vi "data kontrol.vi"() -> ()   [LabVIEW 2021]
panel:
  out "Array 2":dbl[](array[numeric])
  out "Array":dbl[](array[numeric])
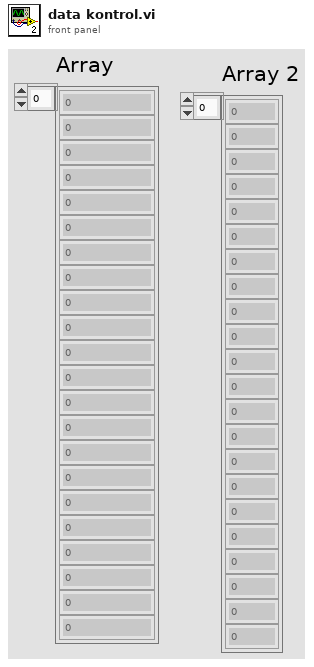
[diagram p1: front panel]
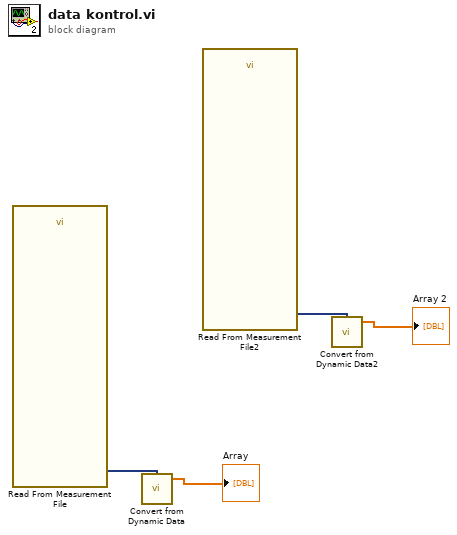
[diagram p0: block diagram]
diagram:
  n1 = call "Read From Measurement File"() -> ("Signals"=w4:dynamicdata)  [unwired: 6 in, 5 out]
  n2 = call "Convert from Dynamic Data"("Dynamic Data Type"=w4) -> ("Array"=→"Array":dbl[])  [unwired: 3 in]
  n3 = call "Read From Measurement File2"() -> ("Signals"=w2:dynamicdata)  [unwired: 6 in, 5 out]
  n4 = call "Convert from Dynamic Data2"("Dynamic Data Type"=w2) -> ("Array"=→"Array 2":dbl[])  [unwired: 3 in]
